vi "parseDataI8.vi"(8 "error in (no error)":errorcluster, 11 "U8ArrayParserAutoIndexing in":refnum<class "U8ArrayParserAutoIndexing.lvclass">) -> (0 "error out":errorcluster, 2 "Data":i8, 3 "U8ArrayParserAutoIndexing out":refnum<class "U8ArrayParserAutoIndexing.lvclass">)   [LabVIEW 2016, in "RTUtilities.lvlib" / "U8ArrayParserAutoIndexing.lvclass"]
uses:
  U8ArrayParserAutoIndexing.lvclass
  U8ArrayParserAutoIndexing.lvclass/U8ArrayParserAutoIndexing.ctl
  U8ArrayParser/U8ArrayParserManualIndexing.lvclass
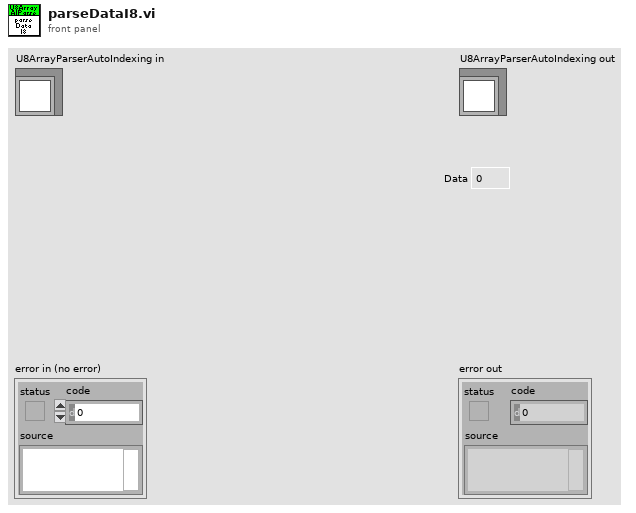
[diagram p1: front panel]
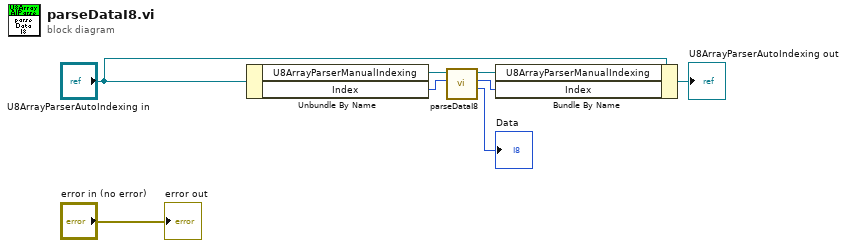
[diagram p0: block diagram]
diagram:
  n1 = Unbundle By Name("U8ArrayParserAutoIndexing in") -> ("U8ArrayParserManualIndexing"=w7:refnum<class "U8ArrayParserManualIndexing.lvclass">, "Index"=w6:i32)
  n2 = call "parseDataI8.vi"("Index"=w6, "U8ArrayParserManualIndexing in"=w7) -> ("Data"=→"Data":i8, "Index out"=w2:i32, "U8ArrayParserManualIndexing out"=w3:refnum<class "U8ArrayParserManualIndexing.lvclass">)  [unwired: 6 in, 1 out]
  n3 = Bundle By Name(cluster="U8ArrayParserAutoIndexing in", "U8ArrayParserManualIndexing"=w3, "Index"=w2) -> (→"U8ArrayParserAutoIndexing out":refnum<class "U8ArrayParserAutoIndexing.lvclass">)
  "error out" <- "error in (no error)"
